vi "save language data.vi"(6 "R/W":enum16{"Read", "Write"}(ring), 8 "error in (no error)":errorcluster, 9 "updated":bool, 10 "Language Data":T1, 11 "appended path":path) -> (0 "error out":errorcluster, 2 "Language Data out":T1)   [LabVIEW 2015, in "AguaClara Library.lvlib"]
uses:
  AguaClara Library.lvlib
  Variable cluster.ctl
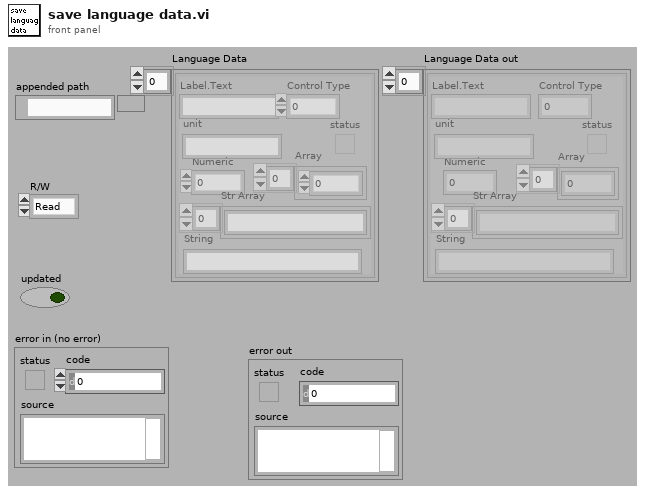
[diagram p1: front panel]
types:
  T1 = typedef "Variable cluster.ctl" = cluster{"Label.Text":string, "Control Type":u32, "Numeric":dbl, "Array":dbl[], "status":bool, "Str Array":string[], "String":string, "unit":string}[]
  T2 = enum16{"open", "replace", "create", "open or create", "replace or create", "replace or create with confirmation"}
  T3 = cluster{"Label.Text":string, "Control Type":u32, "Numeric":dbl, "Array":dbl[], "status":bool, "Str Array":string[], "String":string, "unit":string}
  T4 = cluster{"Label.Text":string, "Control Type":u32, "Numeric":dbl, "Array":dbl[], "status":bool, "Str Array":string[], "String":string, "unit":string}[]
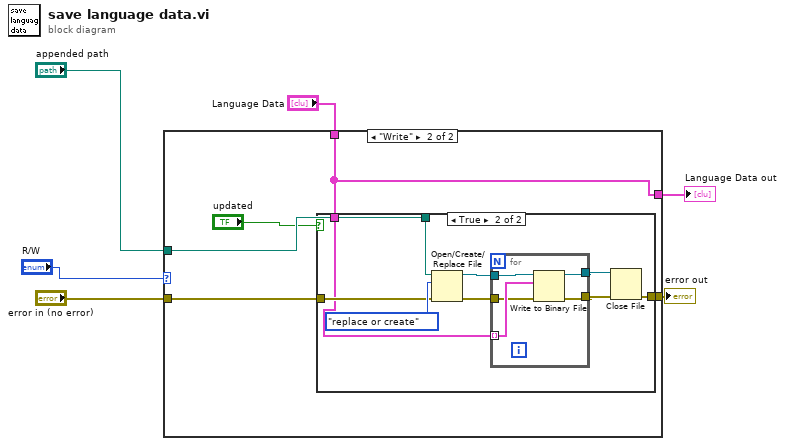
[diagram p0: block diagram]
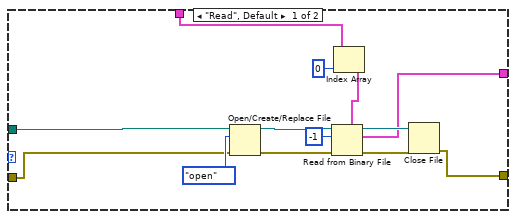
[diagram p2: hidden frame]
diagram:
  n1 = case shown="\"Write\"" "R/W" {
    tunnel: [w10 w24] -> w6
    tunnel: "appended path" -> [w13 w23]
    tunnel: "error in (no error)" -> [w14 w22]
    tunnel: "Language Data" -> [w12 w20]
    tunnel: [w11 w20] -> w2
    frame "Read", Default {
      n2 = Open/Create/Replace File(file path (use dialog)=w13, error in=w14, operation (0:open)=T2."open") -> (refnum out=w15:refnum<file>, error out=w16:errorcluster)  [unwired: 3 in, 1 out]
      n3 = Index Array(array=w12, index=0) -> (element=w8:T3)
      n4 = Read from Binary File(5:w8, 8:w16, 10:-1 ("count"), 11:w15) -> (0:w17:errorcluster, 2:w11:T4, 3:w18:refnum<file>)  [unwired: 2 in, 1 out]
      n5 = Close File(refnum=w18, error in=w17) -> (error out=w10:errorcluster)  [unwired: 1 out]
    }
    frame "Write" {
      n6 = case shown="True" "updated" {
        tunnel: w22 -> [w25 w29]
        tunnel: w23 -> [_ w28]
        tunnel: [w25 w27] -> w24
        tunnel: w20 -> [_ w26]
        frame False {
        }
        frame True {
          n7 = Open/Create/Replace File(file path (use dialog)=w28, error in=w29, operation (0:open)=T2."replace or create") -> (refnum out=w30:refnum<file>, error out=w31:errorcluster)  [unwired: 3 in, 1 out]
          n8 = for {
            tunnel: w30 -> [w39]
            tunnel: [w38] -> w33
            tunnel: [w37] -> w32
            tunnel: w31 -> [w35]
            tunnel: w26 -> [w36] mode=indexing
            n9 = Write to Binary File(file (use dialog)=w39, data=w36, error in=w35) -> (refnum out=w38:refnum<file>, error out=w37:errorcluster)  [unwired: 3 in, 1 out]
          }
          n10 = Close File(refnum=w33, error in=w32) -> (error out=w27:errorcluster)  [unwired: 1 out]
        }
      }
    }
  }
  "error out" <- w6
  "Language Data out" <- w2
